vi "Settings.vi"(11 "Prefs":T2={"Python version"="3.9", "Arduino CLI"=path "", "Python Codes"=[], "Font size"=0, "Text Colors"={"Quote"=46086, "function"=239, "Python"=11817216, "Comment"=15665920, "Triple Quote"=9306312, "Text"=0}, "SSH Logins"=[{"IP Address"="192.168.1.20", "Username"="pi", "password"="password"}]}) -> (3 "Preferences":T1={"python"="", "arduino CLI"=path "", "pythonCodes"=[], "FontSize"=0, "Text Colors"={"Quote"=46086, "function"=239, "Python"=11817216, "Comment"=15665920, "Triple Quote"=9306312, "Text"=0}, "SSH Logins"=[]})   [LabVIEW 2022 SP3]
uses:
  Preferences.ctl
panel:
  in  "TestPython":bool
  in  "update":bool
  # "Welcome to \nME35 Settings"
  # "This program uses python codes under the hood to talk over the serial port, over SSH, and to cameras.  You should using version 3.6 or later and should have pyserial installed."
  # "This dictates the size of the font in the programming area."
  # "This is the path to your Arduino command line interface file - https://www.arduino.cc/pro/cli for more information on how to download and install"
  # "These are the colors used in the python code window."
  # "This is the path to your folder(s) that have all your Python Code (by default, the PythonCode folder on the GitHub, but you can easily change it so that when you update, it does not overwrite that folder)."
  # "Store your Pi login credententials for the ssh connection"
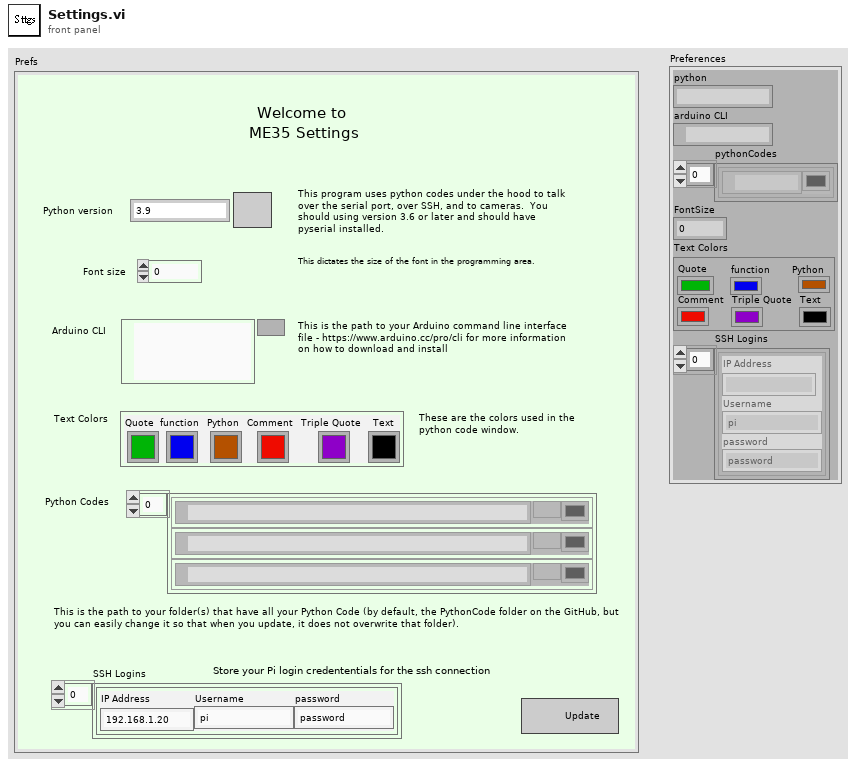
[diagram p1: front panel]
types:
  T1 = typedef "Preferences.ctl" = cluster{"python":string, "arduino CLI":path, "pythonCodes":cluster{"pythonCode":path, "Color":u32}[], "FontSize":u8, "Text Colors":cluster{"Quote":u32, "function":u32, "Python":u32, "Comment":u32, "Triple Quote":u32, "Text":u32}, "SSH Logins":cluster{"IP Address":string, "Username":string, "password":string}[]}
  T2 = cluster{"Python version":string, "Arduino CLI":path, "Python Codes":cluster{"pythonCode":path, "Color":u32}[], "Font size":u8, "Text Colors":cluster{"Quote":u32, "function":u32, "Python":u32, "Comment":u32, "Triple Quote":u32, "Text":u32}, "SSH Logins":cluster{"IP Address":string, "Username":string, "password":string}[]}
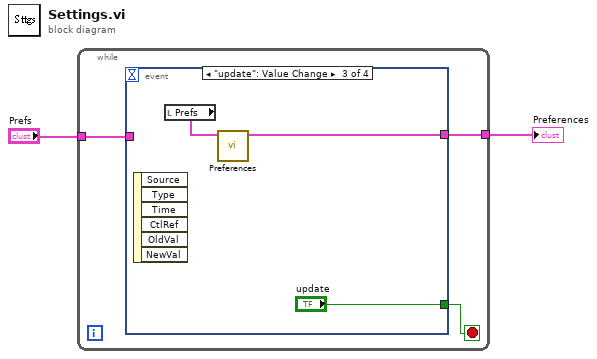
[diagram p0: block diagram]
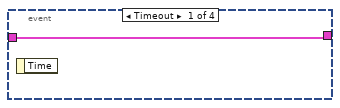
[diagram p2: hidden frame]
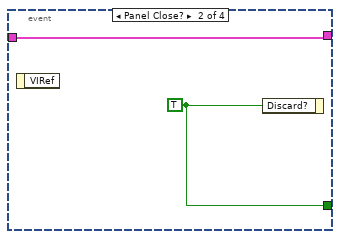
[diagram p3: hidden frame]
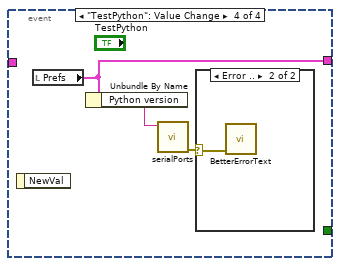
[diagram p4: hidden frame]
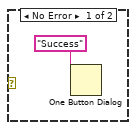
[diagram p5: hidden frame]
diagram:
  n1 = while {
    tunnel: [w4] -> w2
    tunnel: "Prefs" -> [w3]
    stop <- w5 stop-if-true
    n2 = event shown="[2] \"update\": Value Change" {
      selector: _ -> [_ _ _ _]
      dyn-events: _ -> [_ _ _ _]
      timeout: _ -> [_ _ _ _]
      tunnel: [_ w8 "update" _] -> w5
      tunnel: [w6 w7 w10 w14] -> w4
      tunnel: w3 -> [w6 w7 _ _]
      event Timeout {
        n3 = event-data() -> ()  [unwired: 1 in, 1 out]
      }
      event Panel Close? {
        w8 = TRUE ("Discard?")
        n4 = event-data() -> ()  [unwired: 1 in, 1 out]
        n5 = event-data("Discard?"=w8) -> ()  [unwired: 1 in, 1 out]
      }
      event "update": Value Change {
        n6 = event-data() -> ()  [unwired: 1 in, 6 out]
        n7 = local read "Prefs"() -> (w9:T2)
        n8 = call "Preferences.vi"("Preferences in"=w9) -> ("Preferences out"=w10:T1)  [unwired: 9 in, 1 out]
      }
      event "TestPython": Value Change {
        n9 = event-data() -> ()  [unwired: 1 in, 1 out]
        n10 = local read "Prefs"() -> (w14:T2)
        n11 = Unbundle By Name(w14) -> ("Python version"=w13:string)
        n12 = call "serialPorts.vi"("Python version"=w13) -> ("error out"=w12:errorcluster)  [unwired: 7 in, 3 out]
        n13 = case shown="Error .." w12 {
          selector: w12 -> [_ w16]
          frame No Error {
            n14 = One Button Dialog(message="Success") -> ()  [unwired: 1 in, 1 out]
          }
          frame Error {
            n15 = call "BetterErrorText.vi"("error in (no error)"=w16) -> ()  [unwired: 9 in, 2 out]
          }
        }
      }
    }
  }
  "Preferences" <- w2
